vi "sub vi - Read Analog All v9.3.vi"(0 "AI Task0":dbl, 5 "AI Task1":dbl, 7 "AI Task2":dbl) -> (2 "Analog loop time":dbl, 3 "array GRAPH":dynamicdata[](array[waveform]), 4 "LAB01":T2, 6 "LAB02":T3, 8 "LAB03":T4, 10 "LAB04":T5, 13 "deg C":dbl, 14 "USB Error":bool[](array[boolean]), 15 "LAB05":T6)   [LabVIEW 2013]
uses:
  program files/Global display 3.vi
  <vilib>/measure/mascope.llb/Amplitude and Levels 1 chan.vi
  <vilib>/addons/Electrical Power/Basic/Measurement/Power (1 Channel).vi
  <vilib>/addons/Electrical Power/Basic/Measurement/RMS (N Channels).vi
  <vilib>/addons/Electrical Power/Basic/Measurement/RMS (1 Channel).vi
  <vilib>/addons/Electrical Power/Basic/NI_EP_Basic.lvlib
  <vilib>/measure/NI_MAPro.lvlib
panel:
  in  "Tab Control":T1(tab)
  out "LAB01-2 (PF)":dbl
  out "LAB01-1 (PF)":dbl
  out "LAB01-2 (V)":dbl
  out "LAB01-2 (A)":dbl
  out "LAB01-1 (V)":dbl
  out "LAB01-1 (A)":dbl
  out "LAB01-2 (GRAPH)":dynamicdata(graph)
  out "LAB01-1 (GRAPH)":dynamicdata(graph)
  out "LAB02-2 (PF)":dbl
  out "LAB02-1 (PF)":dbl
  out "LAB02-2 (V)":dbl
  out "LAB02-2 (A)":dbl
  out "LAB02-1 (V)":dbl
  out "LAB02-1 (A)":dbl
  out "LAB02-2 (GRAPH)":dynamicdata(graph)
  out "LAB02-1 (GRAPH)":dynamicdata(graph)
  out "LAB03-2 (PF)":dbl
  out "LAB03-1 (PF)":dbl
  out "LAB03-2 (V)":dbl
  out "LAB03-2 (A)":dbl
  out "LAB03-1 (V)":dbl
  out "LAB03-1 (A)":dbl
  out "LAB03-2 (GRAPH)":dynamicdata(graph)
  out "LAB03-1 (GRAPH)":dynamicdata(graph)
  out "LAB04-2 (PF)":dbl
  out "LAB04-1 (PF)":dbl
  out "LAB04-2 (V)":dbl
  out "LAB04-2 (A)":dbl
  out "LAB04-1 (V)":dbl
  out "LAB04-1 (A)":dbl
  out "LAB04-1 (GRAPH)":dynamicdata(graph)
  out "LAB04-2 (GRAPH)":dynamicdata(graph)
  out "LAB05-2 (PF)":dbl
  out "LAB05-1 (PF)":dbl
  out "LAB05-2 (V)":dbl
  out "LAB05-2 (A)":dbl
  out "LAB05-1 (V)":dbl
  out "LAB05-1 (A)":dbl
  out "LAB05-1 (GRAPH)":dynamicdata(graph)
  out "LAB05-2 (GRAPH)":dynamicdata(graph)
  out "A1 error":errorcluster
  out "array ERROR":errorcluster[](array[cluster])
  out "AI2-OFF":waveform(dbl)[](graph)
  out "AI2-ON":waveform(dbl)[](graph)
  out "AI1-OFF":waveform(dbl)[](graph)
  out "AI1-ON":waveform(dbl)[](graph)
  out "AI0-OFF":waveform(dbl)[](graph)
  out "AI0-ON":waveform(dbl)[](graph)
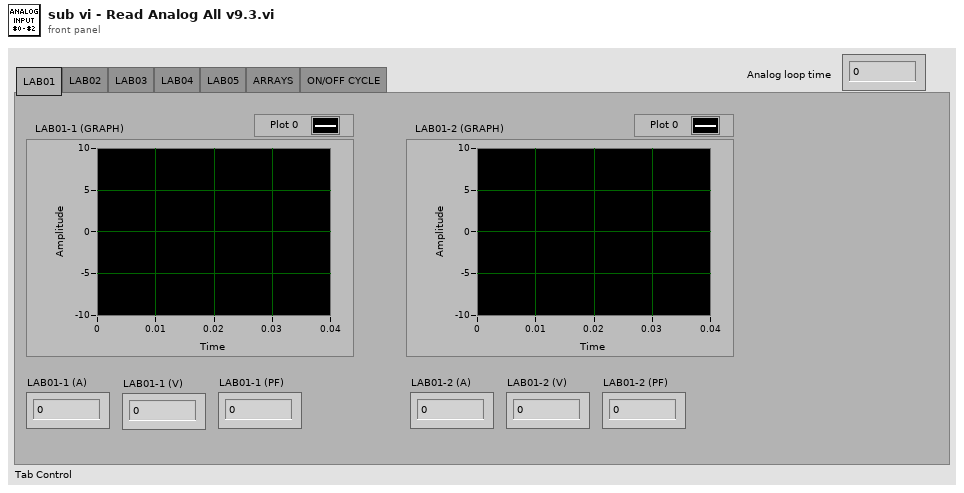
[diagram p1: front panel]
types:
  T1 = enum32{"LAB01", "LAB02", "LAB03", "LAB04", "LAB05", "ARRAYS", "ON/OFF CYCLE"}
  T2 = cluster{"LAB01-1 (A)":dbl, "LAB01-1 (V)":dbl, "LAB01-1 (PF)":dbl, "LAB01-2 (A)":dbl, "LAB01-2 (V)":dbl, "LAB01-2 (PF)":dbl}
  T3 = cluster{"LAB02-1 (A)":dbl, "LAB02-1 (V)":dbl, "LAB02-1 (PF)":dbl, "LAB02-2 (A)":dbl, "LAB02-2 (V)":dbl, "LAB02-2 (PF)":dbl}
  T4 = cluster{"LAB03-1 (A)":dbl, "LAB03-1 (V)":dbl, "LAB03-1 (PF)":dbl, "LAB03-2 (A)":dbl, "LAB03-2 (V)":dbl, "LAB03-2 (PF)":dbl}
  T5 = cluster{"LAB04-1 (A)":dbl, "LAB04-1 (V)":dbl, "LAB04-1 (PF)":dbl, "LAB04-2 (A)":dbl, "LAB04-2 (V)":dbl, "LAB04-2 (PF)":dbl}
  T6 = cluster{"LAB05-1 (A)":dbl, "LAB05-1 (V)":dbl, "LAB05-1 (PF)":dbl, "LAB05-2 (A)":dbl, "LAB05-2 (V)":dbl, "LAB05-2 (PF)":dbl}
  T7 = typedef "NI_EP_Basic.lvlib/basic_Power Value.ctl" = cluster{"active power [W]":dbl, "apparent power [VA]":dbl, "reactive power [VAR]":dbl, "power factor":dbl}
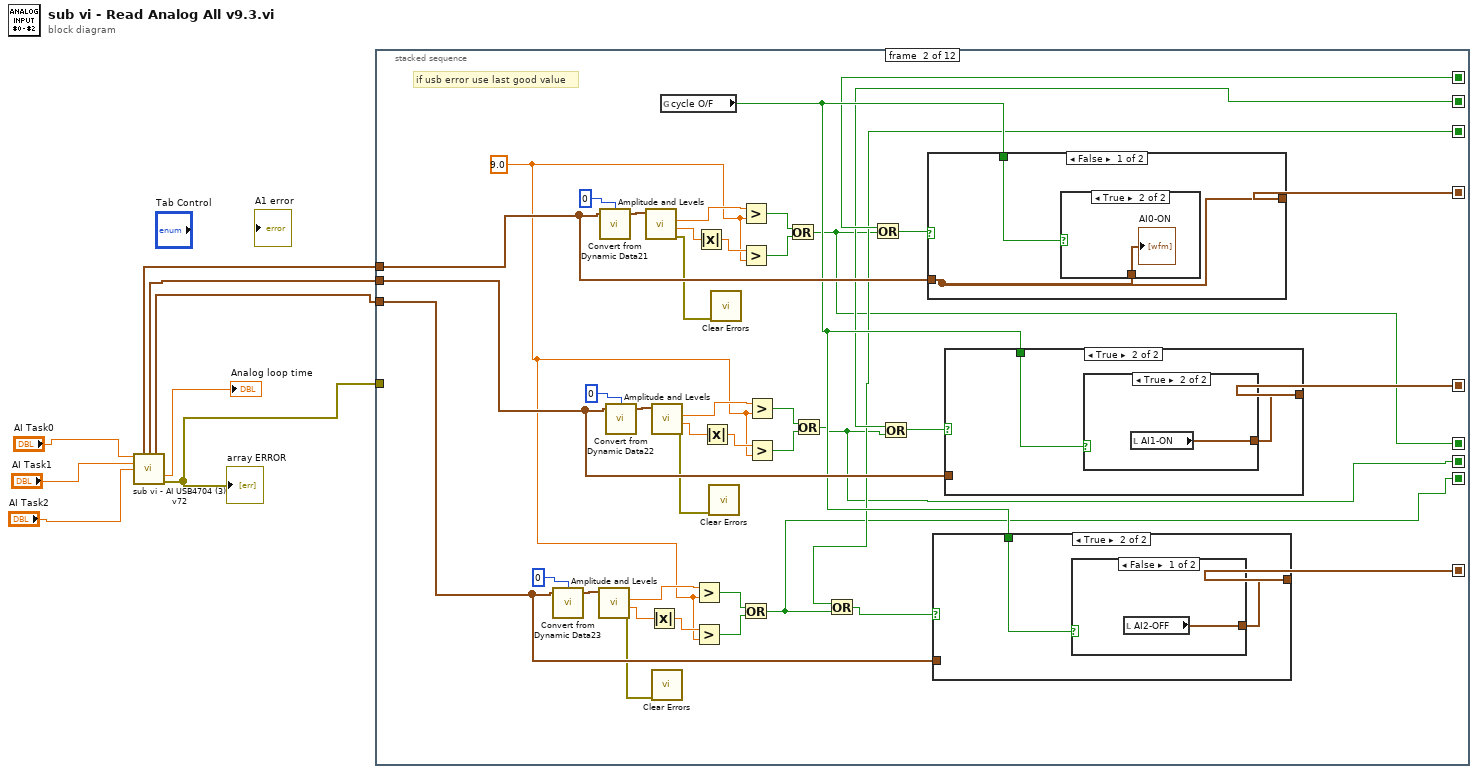
[diagram p0: block diagram]
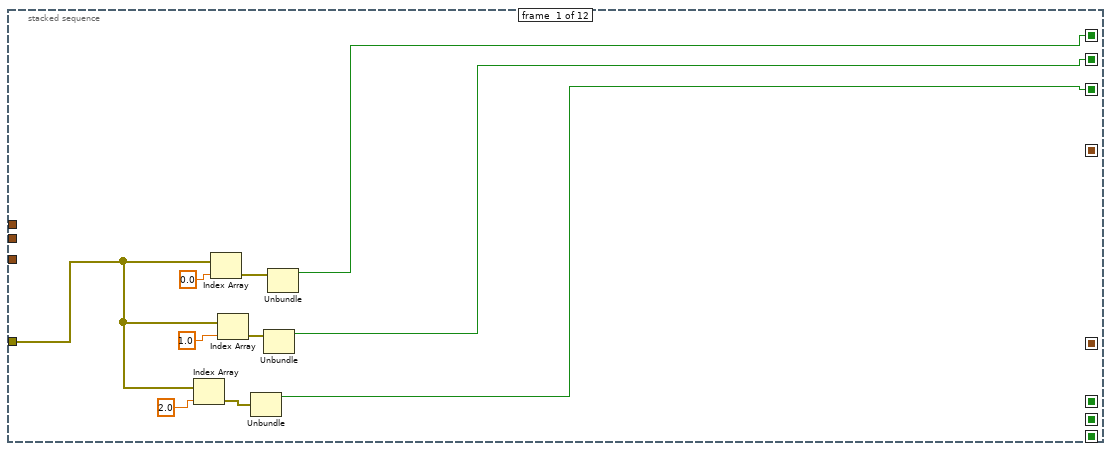
[diagram p2: hidden frame]
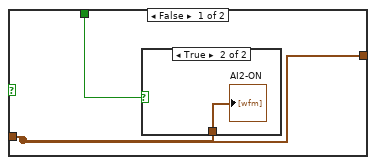
[diagram p3: hidden frame]
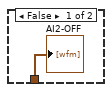
[diagram p4: hidden frame]
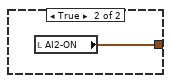
[diagram p5: hidden frame]
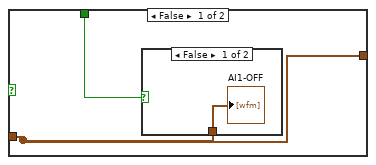
[diagram p6: hidden frame]
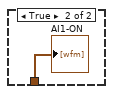
[diagram p7: hidden frame]
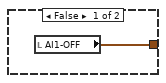
[diagram p8: hidden frame]
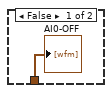
[diagram p9: hidden frame]
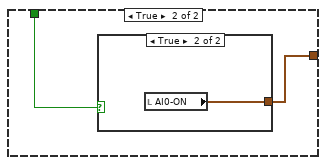
[diagram p10: hidden frame]
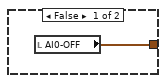
[diagram p11: hidden frame]
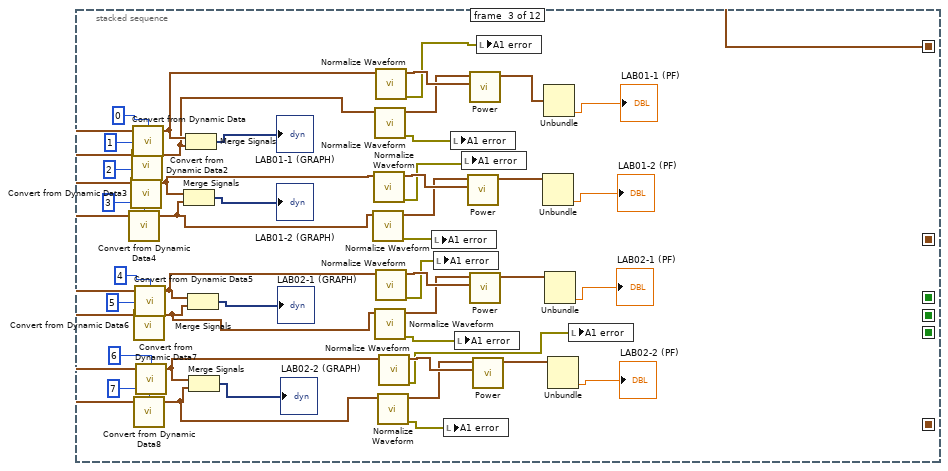
[diagram p12: hidden frame]
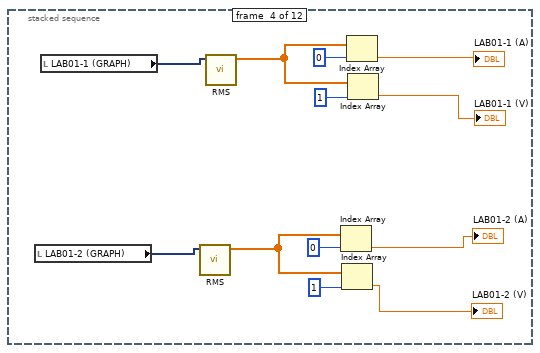
[diagram p13: hidden frame]
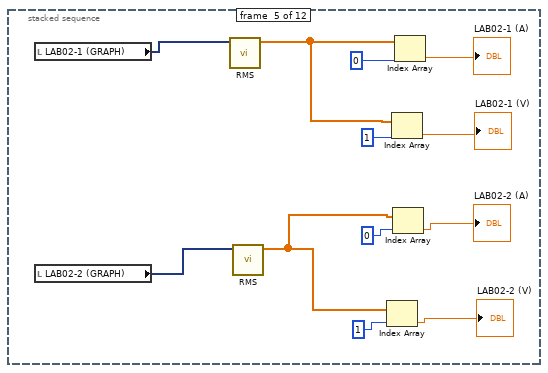
[diagram p14: hidden frame]
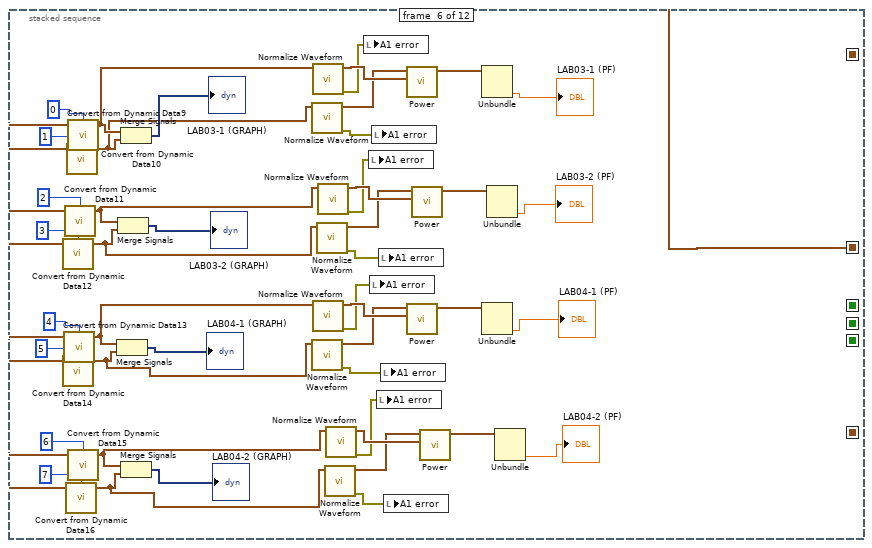
[diagram p15: hidden frame]
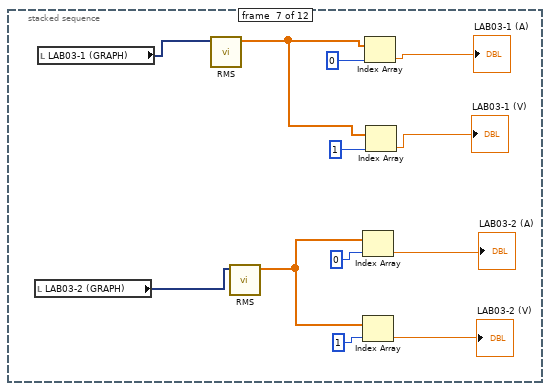
[diagram p16: hidden frame]
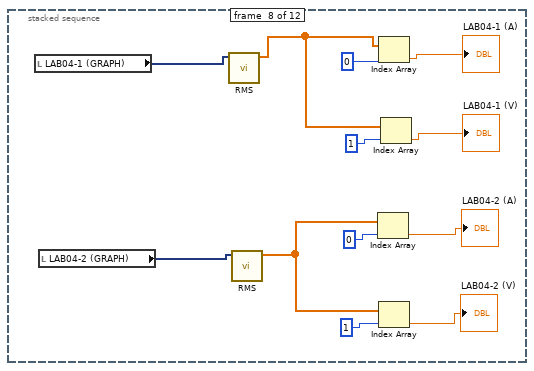
[diagram p17: hidden frame]
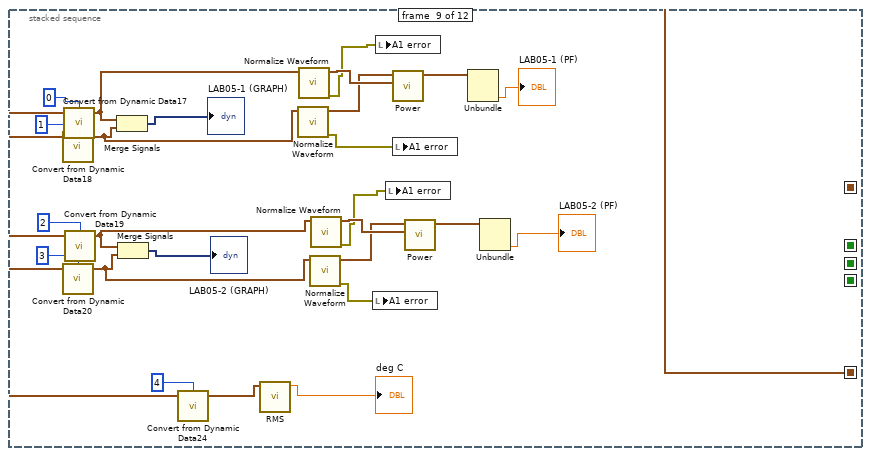
[diagram p18: hidden frame]
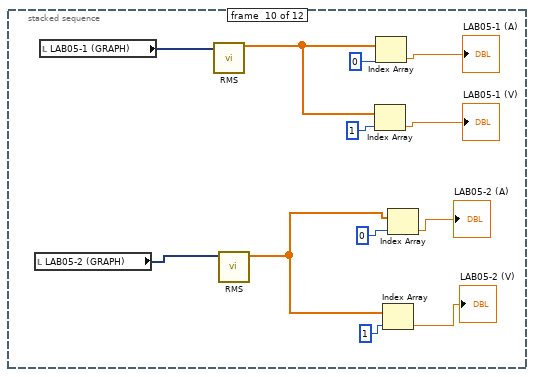
[diagram p19: hidden frame]
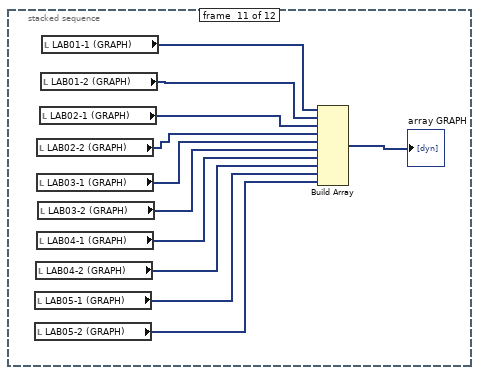
[diagram p20: hidden frame]
diagram:
  n1 = call "sub vi - AI USB4704 (3) v72.vi"("Task0"="AI Task0", "Task1"="AI Task1", "Task2"="AI Task2") -> ("Graph 1"=w8:waveform(dbl)[], "Graph 2"=w7:waveform(dbl)[], "Graph 3"=w6:waveform(dbl)[], "loop time"=→"Analog loop time":dbl, "error array"=w4:errorcluster[])  [unwired: 8 in]
  "array ERROR" <- w4
  n2 = stacked-sequence {
    seq-local: [w16 _ _ _ _ _ _ _ _ _ _ _] -> [_ w26 _ _ _ _ _ _ _ _ _ w276]
    seq-local: [w13 _ _ _ _ _ _ _ _ _ _ _] -> [_ w25 _ _ _ _ _ _ _ _ _ w275]
    seq-local: [w9 _ _ _ _ _ _ _ _ _ _ _] -> [_ w22 _ _ _ _ _ _ _ _ _ w274]
    seq-local: [_ w52 _ _ _ _ _ _ _ _ _ _] -> [_ _ w128 _ _ _ _ _ _ _ _ _]
    seq-local: [_ w42 _ _ _ _ _ _ _ _ _ _] -> [_ _ _ _ _ w197 _ _ _ _ _ _]
    seq-local: [_ w31 _ _ _ _ _ _ _ _ _ _] -> [_ _ _ _ _ _ _ _ w247 _ _ _]
    seq-local: [_ w21 _ _ _ _ _ _ _ _ _ _] -> [_ _ _ _ _ _ _ _ _ _ _ w273]
    seq-local: [_ w20 _ _ _ _ _ _ _ _ _ _] -> [_ _ _ _ _ _ _ _ _ _ _ w272]
    seq-local: [_ w19 _ _ _ _ _ _ _ _ _ _] -> [_ _ _ _ _ _ _ _ _ _ _ w271]
    tunnel: w8 -> [_ w51 _ _ _ _ _ _ _ _ _ _]
    tunnel: w7 -> [_ w43 _ _ _ _ _ _ _ _ _ _]
    tunnel: w6 -> [_ w34 _ _ _ _ _ _ _ _ _ _]
    tunnel: w4 -> [w10 _ _ _ _ _ _ _ _ _ _ _]
    frame #0 {
      n3 = Index Array(array=w10, index=2.0) -> (element=w11:errorcluster)
      n4 = Index Array(array=w10, index=0.0) -> (element=w17:errorcluster)
      n5 = Index Array(array=w10, index=1.0) -> (element=w14:errorcluster)
      n6 = Unbundle(w11) -> ("status"=w9:bool)  [unwired: 2 out]
      n7 = Unbundle(w14) -> ("status"=w13:bool)  [unwired: 2 out]
      n8 = Unbundle(w17) -> ("status"=w16:bool)  [unwired: 2 out]
    }
    frame #1 {
      w33 = 9.0
      # "if usb error use last good value"
      n9 = call "Convert from Dynamic Data23"("Dynamic Data Type"=w34, "Channel"=0) -> ("Waveform"=w40:waveform(dbl))  [unwired: 2 in]
      n10 = call-poly <vilib>:"Amplitude and Levels.vi"("signal in"=w40) -> ("error out"=w28:errorcluster, "low state level"=w39:dbl, "high state level"=w38:dbl)  [unwired: 7 in, 1 out]
      n11 = call "Convert from Dynamic Data21"("Dynamic Data Type"=w51, "Channel"=0) -> ("Waveform"=w58:waveform(dbl))  [unwired: 2 in]
      n12 = call "Convert from Dynamic Data22"("Dynamic Data Type"=w43, "Channel"=0) -> ("Waveform"=w49:waveform(dbl))  [unwired: 2 in]
      n13 = call-poly <vilib>:"Amplitude and Levels.vi"("signal in"=w58) -> ("error out"=w30:errorcluster, "low state level"=w57:dbl, "high state level"=w56:dbl)  [unwired: 7 in, 1 out]
      n14 = Absolute Value(x=w39) -> (abs(x)=w37:dbl)
      n15 = call-poly <vilib>:"Amplitude and Levels.vi"("signal in"=w49) -> ("error out"=w29:errorcluster, "low state level"=w48:dbl, "high state level"=w47:dbl)  [unwired: 7 in, 1 out]
      n16 = call <vilib>:"Clear Errors.vi"("error in (no error)"=w28) -> ()  [unwired: 6 in, 1 out]
      n17 = global read "Global display 3.vi" "cycle O/F"() -> (w32:bool)
      n18 = Greater?(x=w38, y=w33) -> (0:w36:bool)
      n19 = Greater?(x=w37, y=w33) -> (0:w35:bool)
      n20 = Absolute Value(x=w57) -> (abs(x)=w55:dbl)
      n21 = Absolute Value(x=w48) -> (abs(x)=w46:dbl)
      n22 = call <vilib>:"Clear Errors.vi"("error in (no error)"=w29) -> ()  [unwired: 6 in, 1 out]
      n23 = call <vilib>:"Clear Errors.vi"("error in (no error)"=w30) -> ()  [unwired: 6 in, 1 out]
      n24 = Greater?(x=w56, y=w33) -> (0:w54:bool)
      n25 = Greater?(x=w55, y=w33) -> (0:w53:bool)
      n26 = Or(x=w36, y=w35) -> (x .or. y?=w19:bool)
      n27 = Greater?(x=w47, y=w33) -> (0:w45:bool)
      n28 = Greater?(x=w46, y=w33) -> (0:w44:bool)
      n29 = Or(x=w54, y=w53) -> (x .or. y?=w21:bool)
      n30 = Or(x=w45, y=w44) -> (x .or. y?=w20:bool)
      n31 = Or(x=w22, y=w19) -> (x .or. y?=w23:bool)
      n32 = Or(x=w26, y=w21) -> (x .or. y?=w27:bool)
      n33 = Or(x=w25, y=w20) -> (x .or. y?=w24:bool)
      n34 = case shown="False" w27 {
        tunnel: w32 -> [w77 w81]
        tunnel: [w76 w80] -> w52
        tunnel: w51 -> [w76 _]
        frame False {
          n35 = case shown="True" w77 {
            tunnel: w76 -> [w78 w79]
            frame False {
              "AI0-OFF" <- w78
            }
            frame True {
              "AI0-ON" <- w79
            }
          }
        }
        frame True {
          n36 = case shown="True" w81 {
            tunnel: [w82 w83] -> w80
            frame False {
              n37 = local read "AI0-OFF"() -> (w82:waveform(dbl)[])
            }
            frame True {
              n38 = local read "AI0-ON"() -> (w83:waveform(dbl)[])
            }
          }
        }
      }
      n39 = case shown="True" w23 {
        tunnel: w32 -> [w61 w65]
        tunnel: [w60 w64] -> w31
        tunnel: w34 -> [w60 _]
        frame False {
          n40 = case shown="True" w61 {
            tunnel: w60 -> [w62 w63]
            frame False {
              "AI2-OFF" <- w62
            }
            frame True {
              "AI2-ON" <- w63
            }
          }
        }
        frame True {
          n41 = case shown="False" w65 {
            tunnel: [w66 w67] -> w64
            frame False {
              n42 = local read "AI2-OFF"() -> (w66:waveform(dbl)[])
            }
            frame True {
              n43 = local read "AI2-ON"() -> (w67:waveform(dbl)[])
            }
          }
        }
      }
      n44 = case shown="True" w24 {
        tunnel: w32 -> [w69 w73]
        tunnel: [w68 w72] -> w42
        tunnel: w43 -> [w68 _]
        frame False {
          n45 = case shown="False" w69 {
            tunnel: w68 -> [w70 w71]
            frame False {
              "AI1-OFF" <- w70
            }
            frame True {
              "AI1-ON" <- w71
            }
          }
        }
        frame True {
          n46 = case shown="True" w73 {
            tunnel: [w74 w75] -> w72
            frame False {
              n47 = local read "AI1-OFF"() -> (w74:waveform(dbl)[])
            }
            frame True {
              n48 = local read "AI1-ON"() -> (w75:waveform(dbl)[])
            }
          }
        }
      }
    }
    frame #2 {
      n49 = call "Convert from Dynamic Data4"("Dynamic Data Type"=w128, "Channel"=3) -> ("Waveform"=w104:waveform(dbl))  [unwired: 2 in]
      n50 = call "Convert from Dynamic Data3"("Dynamic Data Type"=w128, "Channel"=2) -> ("Waveform"=w105:waveform(dbl))  [unwired: 2 in]
      n51 = call "Convert from Dynamic Data2"("Dynamic Data Type"=w128, "Channel"=1) -> ("Waveform"=w114:waveform(dbl))  [unwired: 2 in]
      n52 = call "Convert from Dynamic Data"("Dynamic Data Type"=w128, "Channel"=0) -> ("Waveform"=w115:waveform(dbl))  [unwired: 2 in]
      n53 = call "Convert from Dynamic Data6"("Dynamic Data Type"=w128, "Channel"=5) -> ("Waveform"=w99:waveform(dbl))  [unwired: 2 in]
      n54 = call "Convert from Dynamic Data8"("Dynamic Data Type"=w128, "Channel"=7) -> ("Waveform"=w93:waveform(dbl))  [unwired: 2 in]
      n55 = call "Convert from Dynamic Data5"("Dynamic Data Type"=w128, "Channel"=4) -> ("Waveform"=w100:waveform(dbl))  [unwired: 2 in]
      n56 = call "Convert from Dynamic Data7"("Dynamic Data Type"=w128, "Channel"=6) -> ("Waveform"=w94:waveform(dbl))  [unwired: 2 in]
      n57 = Merge Signals(w105, w104) -> (→"LAB01-2 (GRAPH)":dynamicdata)
      n58 = Merge Signals(w115, w114) -> (→"LAB01-1 (GRAPH)":dynamicdata)
      n59 = Merge Signals(w100, w99) -> (→"LAB02-1 (GRAPH)":dynamicdata)
      n60 = Merge Signals(w94, w93) -> (→"LAB02-2 (GRAPH)":dynamicdata)
      n61 = call <vilib>:"Normalize Waveform.vi"("waveform in"=w104) -> ("error out"=w88:errorcluster, "normalized waveform"=w108:waveform(dbl))  [unwired: 7 in, 2 out]
      n62 = call <vilib>:"Normalize Waveform.vi"("waveform in"=w105) -> ("error out"=w89:errorcluster, "normalized waveform"=w109:waveform(dbl))  [unwired: 7 in, 2 out]
      n63 = call <vilib>:"Normalize Waveform.vi"("waveform in"=w114) -> ("error out"=w90:errorcluster, "normalized waveform"=w112:waveform(dbl))  [unwired: 7 in, 2 out]
      n64 = call <vilib>:"Normalize Waveform.vi"("waveform in"=w99) -> ("error out"=w86:errorcluster, "normalized waveform"=w102:waveform(dbl))  [unwired: 7 in, 2 out]
      n65 = call <vilib>:"Normalize Waveform.vi"("waveform in"=w115) -> ("error out"=w91:errorcluster, "normalized waveform"=w113:waveform(dbl))  [unwired: 7 in, 2 out]
      n66 = call <vilib>:"Normalize Waveform.vi"("waveform in"=w100) -> ("error out"=w87:errorcluster, "normalized waveform"=w103:waveform(dbl))  [unwired: 7 in, 2 out]
      n67 = call <vilib>:"Normalize Waveform.vi"("waveform in"=w93) -> ("error out"=w84:errorcluster, "normalized waveform"=w96:waveform(dbl))  [unwired: 7 in, 2 out]
      n68 = call <vilib>:"Normalize Waveform.vi"("waveform in"=w94) -> ("error out"=w85:errorcluster, "normalized waveform"=w97:waveform(dbl))  [unwired: 7 in, 2 out]
      n69 = local write "A1 error"(w88) -> ()
      n70 = local write "A1 error"(w87) -> ()
      n71 = local write "A1 error"(w84) -> ()
      n72 = local write "A1 error"(w90) -> ()
      n73 = local write "A1 error"(w86) -> ()
      n74 = local write "A1 error"(w89) -> ()
      n75 = call-poly <vilib>:"Power.vi"("current waveform"=w109, "voltage waveform"=w108) -> ("power value"=w107:T7)  [unwired: 8 in, 1 out]
      n76 = call-poly <vilib>:"Power.vi"("current waveform"=w113, "voltage waveform"=w112) -> ("power value"=w111:T7)  [unwired: 8 in, 1 out]
      n77 = call-poly <vilib>:"Power.vi"("current waveform"=w103, "voltage waveform"=w102) -> ("power value"=w101:T7)  [unwired: 8 in, 1 out]
      n78 = call-poly <vilib>:"Power.vi"("current waveform"=w97, "voltage waveform"=w96) -> ("power value"=w95:T7)  [unwired: 8 in, 1 out]
      n79 = local write "A1 error"(w91) -> ()
      n80 = Unbundle(w107) -> ("power factor"=→"LAB01-2 (PF)":dbl)  [unwired: 3 out]
      n81 = Unbundle(w111) -> ("power factor"=→"LAB01-1 (PF)":dbl)  [unwired: 3 out]
      n82 = Unbundle(w101) -> ("power factor"=→"LAB02-1 (PF)":dbl)  [unwired: 3 out]
      n83 = Unbundle(w95) -> ("power factor"=→"LAB02-2 (PF)":dbl)  [unwired: 3 out]
      n84 = local write "A1 error"(w85) -> ()
    }
    frame #3 {
      n85 = local read "LAB01-2 (GRAPH)"() -> (w137:dynamicdata)
      n86 = local read "LAB01-1 (GRAPH)"() -> (w131:dynamicdata)
      n87 = call-poly <vilib>:"RMS.vi"("waveforms"=w137) -> ("RMS values"=w136:dbl[])  [unwired: 9 in, 1 out]
      n88 = call-poly <vilib>:"RMS.vi"("waveforms"=w131) -> ("RMS values"=w140:dbl[])  [unwired: 9 in, 1 out]
      n89 = Index Array(array=w136, index=0) -> (element=→"LAB01-2 (A)":dbl)
      n90 = Index Array(array=w136, index=1) -> (element=→"LAB01-2 (V)":dbl)
      n91 = Index Array(array=w140, index=0) -> (element=→"LAB01-1 (A)":dbl)
      n92 = Index Array(array=w140, index=1) -> (element=→"LAB01-1 (V)":dbl)
    }
    frame #4 {
      n93 = local read "LAB02-1 (GRAPH)"() -> (w148:dynamicdata)
      n94 = local read "LAB02-2 (GRAPH)"() -> (w144:dynamicdata)
      n95 = call-poly <vilib>:"RMS.vi"("waveforms"=w148) -> ("RMS values"=w147:dbl[])  [unwired: 9 in, 1 out]
      n96 = call-poly <vilib>:"RMS.vi"("waveforms"=w144) -> ("RMS values"=w143:dbl[])  [unwired: 9 in, 1 out]
      n97 = Index Array(array=w143, index=1) -> (element=→"LAB02-2 (V)":dbl)
      n98 = Index Array(array=w147, index=1) -> (element=→"LAB02-1 (V)":dbl)
      n99 = Index Array(array=w143, index=0) -> (element=→"LAB02-2 (A)":dbl)
      n100 = Index Array(array=w147, index=0) -> (element=→"LAB02-1 (A)":dbl)
    }
    frame #5 {
      n101 = call "Convert from Dynamic Data12"("Dynamic Data Type"=w197, "Channel"=3) -> ("Waveform"=w174:waveform(dbl))  [unwired: 2 in]
      n102 = call "Convert from Dynamic Data14"("Dynamic Data Type"=w197, "Channel"=5) -> ("Waveform"=w168:waveform(dbl))  [unwired: 2 in]
      n103 = call "Convert from Dynamic Data13"("Dynamic Data Type"=w197, "Channel"=4) -> ("Waveform"=w169:waveform(dbl))  [unwired: 2 in]
      n104 = call "Convert from Dynamic Data11"("Dynamic Data Type"=w197, "Channel"=2) -> ("Waveform"=w175:waveform(dbl))  [unwired: 2 in]
      n105 = call "Convert from Dynamic Data16"("Dynamic Data Type"=w197, "Channel"=7) -> ("Waveform"=w162:waveform(dbl))  [unwired: 2 in]
      n106 = call "Convert from Dynamic Data10"("Dynamic Data Type"=w197, "Channel"=1) -> ("Waveform"=w180:waveform(dbl))  [unwired: 2 in]
      n107 = call "Convert from Dynamic Data9"("Dynamic Data Type"=w197, "Channel"=0) -> ("Waveform"=w181:waveform(dbl))  [unwired: 2 in]
      n108 = call "Convert from Dynamic Data15"("Dynamic Data Type"=w197, "Channel"=6) -> ("Waveform"=w163:waveform(dbl))  [unwired: 2 in]
      n109 = Merge Signals(w169, w168) -> (→"LAB04-1 (GRAPH)":dynamicdata)
      n110 = Merge Signals(w175, w174) -> (→"LAB03-2 (GRAPH)":dynamicdata)
      n111 = Merge Signals(w181, w180) -> (→"LAB03-1 (GRAPH)":dynamicdata)
      n112 = Merge Signals(w163, w162) -> (→"LAB04-2 (GRAPH)":dynamicdata)
      n113 = call <vilib>:"Normalize Waveform.vi"("waveform in"=w180) -> ("error out"=w159:errorcluster, "normalized waveform"=w183:waveform(dbl))  [unwired: 7 in, 2 out]
      n114 = call <vilib>:"Normalize Waveform.vi"("waveform in"=w168) -> ("error out"=w155:errorcluster, "normalized waveform"=w171:waveform(dbl))  [unwired: 7 in, 2 out]
      n115 = call <vilib>:"Normalize Waveform.vi"("waveform in"=w181) -> ("error out"=w160:errorcluster, "normalized waveform"=w184:waveform(dbl))  [unwired: 7 in, 2 out]
      n116 = call <vilib>:"Normalize Waveform.vi"("waveform in"=w169) -> ("error out"=w156:errorcluster, "normalized waveform"=w172:waveform(dbl))  [unwired: 7 in, 2 out]
      n117 = call <vilib>:"Normalize Waveform.vi"("waveform in"=w174) -> ("error out"=w157:errorcluster, "normalized waveform"=w177:waveform(dbl))  [unwired: 7 in, 2 out]
      n118 = call <vilib>:"Normalize Waveform.vi"("waveform in"=w175) -> ("error out"=w158:errorcluster, "normalized waveform"=w178:waveform(dbl))  [unwired: 7 in, 2 out]
      n119 = call <vilib>:"Normalize Waveform.vi"("waveform in"=w162) -> ("error out"=w153:errorcluster, "normalized waveform"=w165:waveform(dbl))  [unwired: 7 in, 2 out]
      n120 = call <vilib>:"Normalize Waveform.vi"("waveform in"=w163) -> ("error out"=w154:errorcluster, "normalized waveform"=w166:waveform(dbl))  [unwired: 7 in, 2 out]
      n121 = local write "A1 error"(w160) -> ()
      n122 = local write "A1 error"(w158) -> ()
      n123 = local write "A1 error"(w156) -> ()
      n124 = local write "A1 error"(w159) -> ()
      n125 = local write "A1 error"(w154) -> ()
      n126 = local write "A1 error"(w157) -> ()
      n127 = local write "A1 error"(w155) -> ()
      n128 = local write "A1 error"(w153) -> ()
      n129 = call-poly <vilib>:"Power.vi"("current waveform"=w184, "voltage waveform"=w183) -> ("power value"=w182:T7)  [unwired: 8 in, 1 out]
      n130 = call-poly <vilib>:"Power.vi"("current waveform"=w172, "voltage waveform"=w171) -> ("power value"=w170:T7)  [unwired: 8 in, 1 out]
      n131 = call-poly <vilib>:"Power.vi"("current waveform"=w178, "voltage waveform"=w177) -> ("power value"=w176:T7)  [unwired: 8 in, 1 out]
      n132 = call-poly <vilib>:"Power.vi"("current waveform"=w166, "voltage waveform"=w165) -> ("power value"=w164:T7)  [unwired: 8 in, 1 out]
      n133 = Unbundle(w182) -> ("power factor"=→"LAB03-1 (PF)":dbl)  [unwired: 3 out]
      n134 = Unbundle(w170) -> ("power factor"=→"LAB04-1 (PF)":dbl)  [unwired: 3 out]
      n135 = Unbundle(w176) -> ("power factor"=→"LAB03-2 (PF)":dbl)  [unwired: 3 out]
      n136 = Unbundle(w164) -> ("power factor"=→"LAB04-2 (PF)":dbl)  [unwired: 3 out]
    }
    frame #6 {
      n137 = local read "LAB03-2 (GRAPH)"() -> (w204:dynamicdata)
      n138 = local read "LAB03-1 (GRAPH)"() -> (w205:dynamicdata)
      n139 = call-poly <vilib>:"RMS.vi"("waveforms"=w205) -> ("RMS values"=w203:dbl[])  [unwired: 9 in, 1 out]
      n140 = call-poly <vilib>:"RMS.vi"("waveforms"=w204) -> ("RMS values"=w200:dbl[])  [unwired: 9 in, 1 out]
      n141 = Index Array(array=w200, index=0) -> (element=→"LAB03-2 (A)":dbl)
      n142 = Index Array(array=w200, index=1) -> (element=→"LAB03-2 (V)":dbl)
      n143 = Index Array(array=w203, index=0) -> (element=→"LAB03-1 (A)":dbl)
      n144 = Index Array(array=w203, index=1) -> (element=→"LAB03-1 (V)":dbl)
    }
    frame #7 {
      n145 = local read "LAB04-1 (GRAPH)"() -> (w217:dynamicdata)
      n146 = local read "LAB04-2 (GRAPH)"() -> (w213:dynamicdata)
      n147 = call-poly <vilib>:"RMS.vi"("waveforms"=w217) -> ("RMS values"=w216:dbl[])  [unwired: 9 in, 1 out]
      n148 = call-poly <vilib>:"RMS.vi"("waveforms"=w213) -> ("RMS values"=w212:dbl[])  [unwired: 9 in, 1 out]
      n149 = Index Array(array=w212, index=0) -> (element=→"LAB04-2 (A)":dbl)
      n150 = Index Array(array=w216, index=0) -> (element=→"LAB04-1 (A)":dbl)
      n151 = Index Array(array=w212, index=1) -> (element=→"LAB04-2 (V)":dbl)
      n152 = Index Array(array=w216, index=1) -> (element=→"LAB04-1 (V)":dbl)
    }
    frame #8 {
      n153 = call "Convert from Dynamic Data18"("Dynamic Data Type"=w247, "Channel"=1) -> ("Waveform"=w236:waveform(dbl))  [unwired: 2 in]
      n154 = call "Convert from Dynamic Data20"("Dynamic Data Type"=w247, "Channel"=3) -> ("Waveform"=w230:waveform(dbl))  [unwired: 2 in]
      n155 = call "Convert from Dynamic Data17"("Dynamic Data Type"=w247, "Channel"=0) -> ("Waveform"=w237:waveform(dbl))  [unwired: 2 in]
      n156 = call "Convert from Dynamic Data19"("Dynamic Data Type"=w247, "Channel"=2) -> ("Waveform"=w231:waveform(dbl))  [unwired: 2 in]
      n157 = Merge Signals(w237, w236) -> (→"LAB05-1 (GRAPH)":dynamicdata)
      n158 = Merge Signals(w231, w230) -> (→"LAB05-2 (GRAPH)":dynamicdata)
      n159 = call "Convert from Dynamic Data24"("Dynamic Data Type"=w247, "Channel"=4) -> ("Waveform"=w223:waveform(dbl))  [unwired: 2 in]
      n160 = call-poly <vilib>:"RMS.vi"("waveform"=w223) -> ("RMS value"=→"deg C":dbl)  [unwired: 9 in, 1 out]
      n161 = call <vilib>:"Normalize Waveform.vi"("waveform in"=w236) -> ("error out"=w228:errorcluster, "normalized waveform"=w239:waveform(dbl))  [unwired: 7 in, 2 out]
      n162 = call <vilib>:"Normalize Waveform.vi"("waveform in"=w237) -> ("error out"=w227:errorcluster, "normalized waveform"=w240:waveform(dbl))  [unwired: 7 in, 2 out]
      n163 = call <vilib>:"Normalize Waveform.vi"("waveform in"=w230) -> ("error out"=w226:errorcluster, "normalized waveform"=w233:waveform(dbl))  [unwired: 7 in, 2 out]
      n164 = call <vilib>:"Normalize Waveform.vi"("waveform in"=w231) -> ("error out"=w225:errorcluster, "normalized waveform"=w234:waveform(dbl))  [unwired: 7 in, 2 out]
      n165 = local write "A1 error"(w226) -> ()
      n166 = local write "A1 error"(w227) -> ()
      n167 = local write "A1 error"(w225) -> ()
      n168 = call-poly <vilib>:"Power.vi"("current waveform"=w240, "voltage waveform"=w239) -> ("power value"=w238:T7)  [unwired: 8 in, 1 out]
      n169 = local write "A1 error"(w228) -> ()
      n170 = call-poly <vilib>:"Power.vi"("current waveform"=w234, "voltage waveform"=w233) -> ("power value"=w232:T7)  [unwired: 8 in, 1 out]
      n171 = Unbundle(w238) -> ("power factor"=→"LAB05-1 (PF)":dbl)  [unwired: 3 out]
      n172 = Unbundle(w232) -> ("power factor"=→"LAB05-2 (PF)":dbl)  [unwired: 3 out]
    }
    frame #9 {
      n173 = local read "LAB05-2 (GRAPH)"() -> (w254:dynamicdata)
      n174 = local read "LAB05-1 (GRAPH)"() -> (w255:dynamicdata)
      n175 = call-poly <vilib>:"RMS.vi"("waveforms"=w255) -> ("RMS values"=w253:dbl[])  [unwired: 9 in, 1 out]
      n176 = call-poly <vilib>:"RMS.vi"("waveforms"=w254) -> ("RMS values"=w252:dbl[])  [unwired: 9 in, 1 out]
      n177 = Index Array(array=w253, index=1) -> (element=→"LAB05-1 (V)":dbl)
      n178 = Index Array(array=w253, index=0) -> (element=→"LAB05-1 (A)":dbl)
      n179 = Index Array(array=w252, index=1) -> (element=→"LAB05-2 (V)":dbl)
      n180 = Index Array(array=w252, index=0) -> (element=→"LAB05-2 (A)":dbl)
    }
    frame #10 {
      n181 = local read "LAB05-1 (GRAPH)"() -> (w262:dynamicdata)
      n182 = local read "LAB05-2 (GRAPH)"() -> (w261:dynamicdata)
      n183 = local read "LAB04-2 (GRAPH)"() -> (w263:dynamicdata)
      n184 = local read "LAB02-2 (GRAPH)"() -> (w267:dynamicdata)
      n185 = local read "LAB03-1 (GRAPH)"() -> (w266:dynamicdata)
      n186 = local read "LAB04-1 (GRAPH)"() -> (w264:dynamicdata)
      n187 = local read "LAB03-2 (GRAPH)"() -> (w265:dynamicdata)
      n188 = local read "LAB02-1 (GRAPH)"() -> (w268:dynamicdata)
      n189 = local read "LAB01-2 (GRAPH)"() -> (w269:dynamicdata)
      n190 = local read "LAB01-1 (GRAPH)"() -> (w270:dynamicdata)
      n191 = Build Array(w270, w269, w268, w267, w266, w265, w264, w263, w262, w261) -> (→"array GRAPH":dynamicdata[])
    }
    frame #11 {
      n192 = local read "LAB03-2 (PF)"() -> (w295:dbl)
      n193 = local read "LAB03-1 (PF)"() -> (w298:dbl)
      n194 = local read "LAB03-1 (A)"() -> (w300:dbl)
      n195 = local read "LAB03-1 (V)"() -> (w299:dbl)
      n196 = local read "LAB03-2 (A)"() -> (w297:dbl)
      n197 = local read "LAB03-2 (V)"() -> (w296:dbl)
      n198 = local read "LAB01-1 (PF)"() -> (w305:dbl)
      n199 = local read "LAB01-2 (PF)"() -> (w302:dbl)
      n200 = local read "LAB01-1 (V)"() -> (w306:dbl)
      n201 = local read "LAB01-2 (A)"() -> (w304:dbl)
      n202 = local read "LAB01-2 (V)"() -> (w303:dbl)
      n203 = local read "LAB01-1 (A)"() -> (w307:dbl)
      n204 = Bundle("LAB03-1 (A)"=w300, "LAB03-1 (V)"=w299, "LAB03-1 (PF)"=w298, "LAB03-2 (A)"=w297, "LAB03-2 (V)"=w296, "LAB03-2 (PF)"=w295) -> (→"LAB03":T4)  [unwired: 1 in]
      n205 = local read "LAB05-2 (PF)"() -> (w281:dbl)
      n206 = local read "LAB05-1 (PF)"() -> (w284:dbl)
      n207 = Bundle("LAB01-1 (A)"=w307, "LAB01-1 (V)"=w306, "LAB01-1 (PF)"=w305, "LAB01-2 (A)"=w304, "LAB01-2 (V)"=w303, "LAB01-2 (PF)"=w302) -> (→"LAB01":T2)  [unwired: 1 in]
      n208 = local read "LAB05-2 (V)"() -> (w282:dbl)
      n209 = local read "LAB05-1 (A)"() -> (w286:dbl)
      n210 = local read "LAB05-1 (V)"() -> (w285:dbl)
      n211 = local read "LAB05-2 (A)"() -> (w283:dbl)
      n212 = local read "LAB04-1 (PF)"() -> (w292:dbl)
      n213 = local read "LAB04-2 (PF)"() -> (w289:dbl)
      n214 = local read "LAB04-1 (A)"() -> (w294:dbl)
      n215 = local read "LAB04-1 (V)"() -> (w293:dbl)
      n216 = local read "LAB04-2 (A)"() -> (w291:dbl)
      n217 = local read "LAB04-2 (V)"() -> (w290:dbl)
      n218 = local read "LAB02-2 (PF)"() -> (w309:dbl)
      n219 = local read "LAB02-1 (PF)"() -> (w312:dbl)
      n220 = local read "LAB02-2 (A)"() -> (w311:dbl)
      n221 = local read "LAB02-2 (V)"() -> (w310:dbl)
      n222 = local read "LAB02-1 (V)"() -> (w313:dbl)
      n223 = local read "LAB02-1 (A)"() -> (w314:dbl)
      n224 = Bundle("LAB05-1 (A)"=w286, "LAB05-1 (V)"=w285, "LAB05-1 (PF)"=w284, "LAB05-2 (A)"=w283, "LAB05-2 (V)"=w282, "LAB05-2 (PF)"=w281) -> (→"LAB05":T6)  [unwired: 1 in]
      n225 = Bundle("LAB04-1 (A)"=w294, "LAB04-1 (V)"=w293, "LAB04-1 (PF)"=w292, "LAB04-2 (A)"=w291, "LAB04-2 (V)"=w290, "LAB04-2 (PF)"=w289) -> (→"LAB04":T5)  [unwired: 1 in]
      n226 = Bundle("LAB02-1 (A)"=w314, "LAB02-1 (V)"=w313, "LAB02-1 (PF)"=w312, "LAB02-2 (A)"=w311, "LAB02-2 (V)"=w310, "LAB02-2 (PF)"=w309) -> (→"LAB02":T3)  [unwired: 1 in]
      n227 = Or(x=w275, y=w272) -> (x .or. y?=w277:bool)
      n228 = Or(x=w276, y=w271) -> (x .or. y?=w279:bool)
      n229 = Or(x=w274, y=w273) -> (x .or. y?=w278:bool)
      n230 = Build Array(w279, w277, w278) -> (→"USB Error":bool[])
    }
  }
